vi "FGVRaceConditionExample.vi"() -> ()   [LabVIEW 2020]
doc: "Example of race condtion with parrarel use FGV with action engine and without. Comments in Polish."
panel:
  out "Out":i32
  in  "In":i32
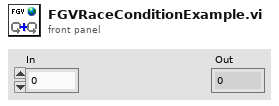
[diagram p1: front panel]
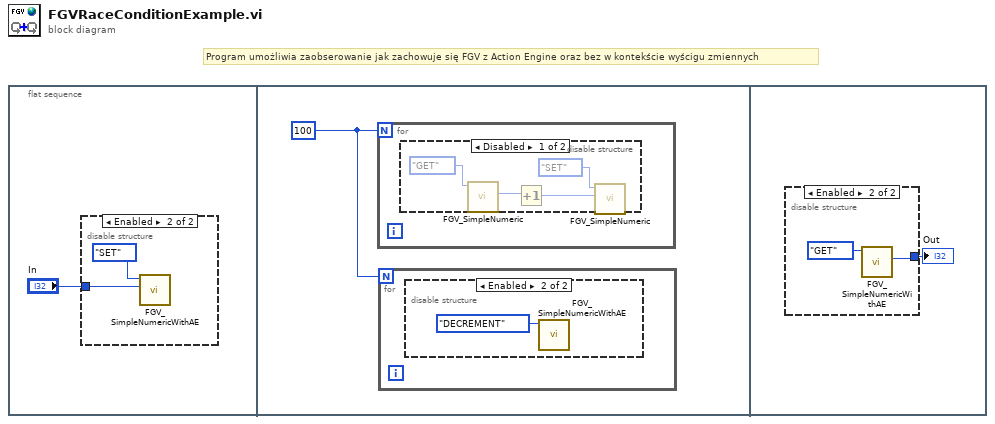
[diagram p0: block diagram]
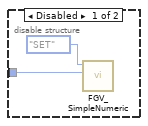
[diagram p2: hidden frame]
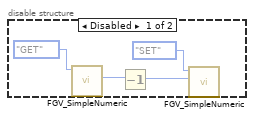
[diagram p3: hidden frame]
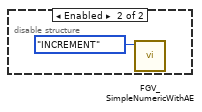
[diagram p4: hidden frame]
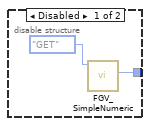
[diagram p5: hidden frame]
diagram:
  # "Program umożliwia zaobserowanie jak zachowuje się FGV z Action Engine oraz bez w kontekście wyścigu zmiennych"
  n1 = flat-sequence {
    frame #0 {
      n2 = disable-structure shown="Enabled" {
        disable-tunnel: "In" -> [w2 w5]
        frame Disabled {
          n3 = call "FGV_SimpleNumeric.vi"("Numeric"=w2, "Mode"=enum16{"SET", "GET"}."SET") -> ()  [unwired: 9 in, 1 out]
        }
        frame Enabled {
          n4 = call "FGV_SimpleNumericWithAE.vi"("Numeric"=w5, "Mode"=enum16{"SET", "GET", "INCREMENT", "DECREMENT"}."SET") -> ()  [unwired: 9 in, 1 out]
        }
      }
    }
    frame #1 {
      w6 = 100
      n5 = for {
        N: w6 -> [_]
        n6 = disable-structure shown="Disabled" {
          frame Disabled {
            n7 = call "FGV_SimpleNumeric.vi"("Mode"=enum16{"SET", "GET"}."GET") -> ("Numeric Out"=w14:i32)  [unwired: 10 in]
            n8 = Increment(x=w14) -> (x+1=w12:i32)
            n9 = call "FGV_SimpleNumeric.vi"("Numeric"=w12, "Mode"=enum16{"SET", "GET"}."SET") -> ()  [unwired: 9 in, 1 out]
          }
          frame Enabled {
            n10 = call "FGV_SimpleNumericWithAE.vi"("Mode"=enum16{"SET", "GET", "INCREMENT", "DECREMENT"}."INCREMENT") -> ()  [unwired: 10 in, 1 out]
          }
        }
      }
      n11 = for {
        N: w6 -> [_]
        n12 = disable-structure shown="Enabled" {
          frame Disabled {
            n13 = call "FGV_SimpleNumeric.vi"("Mode"=enum16{"SET", "GET"}."GET") -> ("Numeric Out"=w8:i32)  [unwired: 10 in]
            n14 = Decrement(x=w8) -> (x-1=w10:i32)
            n15 = call "FGV_SimpleNumeric.vi"("Numeric"=w10, "Mode"=enum16{"SET", "GET"}."SET") -> ()  [unwired: 9 in, 1 out]
          }
          frame Enabled {
            n16 = call "FGV_SimpleNumericWithAE.vi"("Mode"=enum16{"SET", "GET", "INCREMENT", "DECREMENT"}."DECREMENT") -> ()  [unwired: 10 in, 1 out]
          }
        }
      }
    }
    frame #2 {
      n17 = disable-structure shown="Enabled" {
        disable-tunnel: [w19 w21] -> w17
        frame Disabled {
          n18 = call "FGV_SimpleNumeric.vi"("Mode"=enum16{"SET", "GET"}."GET") -> ("Numeric Out"=w19:i32)  [unwired: 10 in]
        }
        frame Enabled {
          n19 = call "FGV_SimpleNumericWithAE.vi"("Mode"=enum16{"SET", "GET", "INCREMENT", "DECREMENT"}."GET") -> ("Numeric Out"=w21:i32)  [unwired: 10 in]
        }
      }
      "Out" <- w17
    }
  }
